vi "cont_acq_voltage_ext.vi"() -> ()   [LabVIEW 2017]
doc: "I. Description:\nThis example demonstrates how to acquire a continuous amount of data (Waveform) using an external sample clock, started by a digital edge.\n\nII. Instructions for Running:\n1. Select the physical channel to correspond to where your signal is input on the DAQ device.\n2. Enter the minimum and maximum voltage ranges.\nNote: For better accuracy try to match the Input Ranges to the expected voltage level of the measured signal.\n3. Select a source for the sample clock.\n4. Set the approximate Rate of the external clock. This allows the internal characteristics of the acquisition to be as efficient as possible. Also set the Samples to Read control. This will determine how many samples are read each time the while loop iterates. This also determines how many points are plotted on the graph each iteration.\n5. Select a source for the digital edge start trigger.\n6. Select the edge, rising or falling, on which to trigger.\n\nIII. Block Diagram Steps:\n1. Create an analog input voltage channel.\n2. Define the parameters for an External Clock Source. Additionally, define the sample mode to be continuous. The external clock rate is given to allow the internal characteristics of the acquisition to be as efficient as possible. \n3. Set the parameters for a digital edge start trigger.\n4. Call the Start VI to start the acquisition.\n5. Read the waveform data in a loop until the user hits the stop button or an error occurs.\nNote: This example reads data from one or more channels and returns an array of data. Use the Index Array function to access an individual channel of data.\n6. Call the Clear Task VI to clear the Task.\n7. Use the popup dialog box to display an error or warning if any.\n\nIV. I/O Connections Overview:\nMake sure your signal input terminal matches the Physical Channel I/O control. Also, make sure your external clock terminal matches the Clock Source Control. Finally, make sure that your digital trigger signal is connected to the terminal specified in Trigger Source. For further connection information, refer to your hardware reference manual."
uses:
  <vilib>/Utility/error.llb/DialogType.ctl
  <vilib>/DAQmx/read.llb/DAQmx Read (Analog 1D Wfm NChan NSamp).vi
  <vilib>/DAQmx/create/channels.llb/DAQmx Create Channel (AI-Voltage-Basic).vi
  <vilib>/DAQmx/configure/timing.llb/DAQmx Timing (Sample Clock).vi
  <vilib>/DAQmx/configure/trigger.llb/DAQmx Start Trigger (Digital Edge).vi
  <vilib>/DAQmx/miscellaneous.llb/DAQmx Fill In Error Info.vi
panel:
  in  "Samples to Read":i32=1000
  in  "Trigger Edge":i32(ring)=10280 items=["Rising"=10280, "Falling"=10171]
  in  "Trigger Source":tag="/Dev1/PFI0"
  in  "Maximum Value":dbl=10.0 format="%0.2f"
  in  "Minimum Value":dbl=-10.0 format="%0.2f"
  in  "Physical Channel":tag="Dev1/ai0"
  in  "Rate":dbl=10000.0 caption="Sample Rate (Hz)" format="%0.2f"
  in  "Clock Source":tag="/Dev1/PFI7"
  in  "stop":bool
  out "Measurement":waveform(dbl)[](graph)
  # "For instructions, select Help>>Show Context Help"
  # "Channel Parameters"
  # "Timing Parameters"
  # "Trigger Parameters"
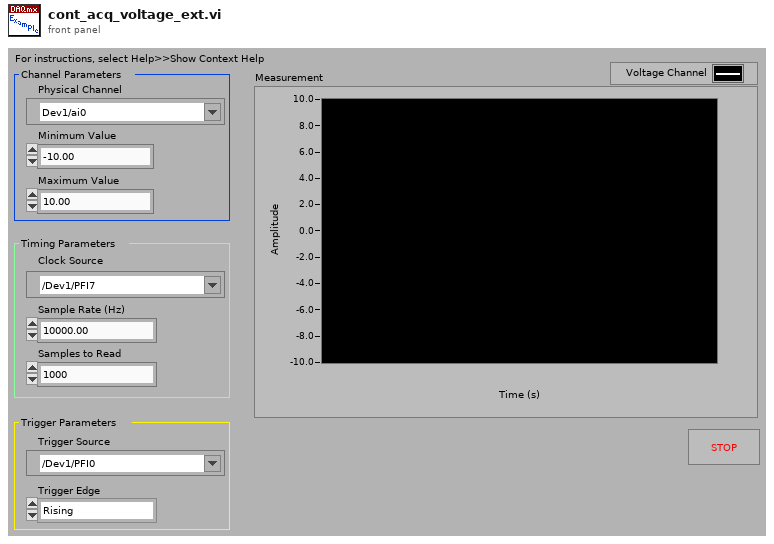
[diagram p1: front panel]
types:
  T1 = typedef "DialogType.ctl" = u16
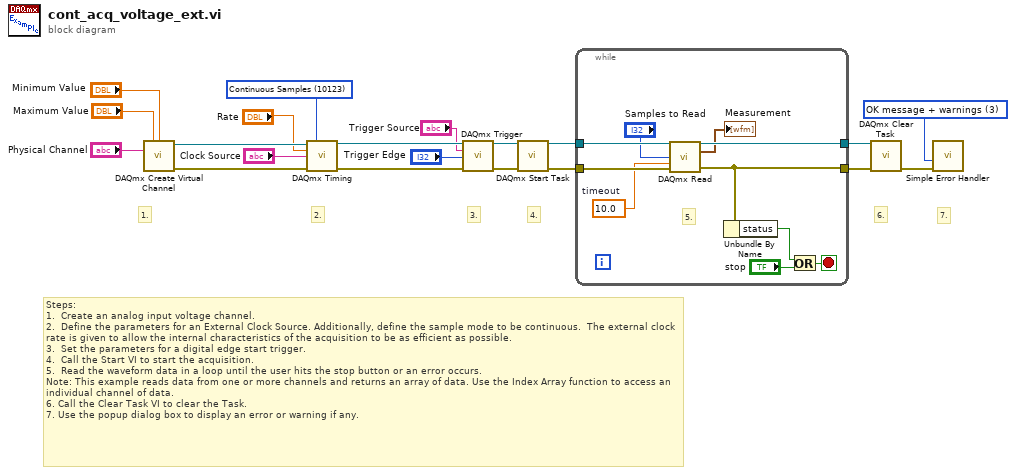
[diagram p0: block diagram]
diagram:
  w3 = T1 3 items=["no dialog", "OK message", "continue or stop message", "OK message + warnings", "continue/stop + warnings"] ("type of dialog (OK msg:1)")
  w7 = 10123 items=["Finite Samples"=10178, "Continuous Samples"=10123] ("sample mode")
  # "7."
  # "Steps: \n1.  Create an analog input voltage channel.\n2.  Define the parameters for an External Clock Source. Additionally, define the sample mode to be continuous.  The external clock rate is given to allow the internal characteristics of the acquisition to be as efficient as possible.  \n3.  Set the parameters for a digital edge start trigger.\n4.  Call the Start VI to start the acquisition.\n5.  Read the waveform data in a loop until the user hits the stop button or an error occurs.\nNote: This example reads data from one or more channels and returns an array of data. Use the Index Array function to access an individual channel of data.\n6. Call the Clear Task VI to clear the Task.\n7. Use the popup dialog box to display an error or warning if any."
  # "6."
  # "4."
  # "3."
  # "2."
  # "1."
  n1 = call-poly <vilib>:"DAQmx Create Virtual Channel.vi"("maximum value"="Maximum Value", "minimum value"="Minimum Value", "physical channels"="Physical Channel") -> ("task out"=w13:refnum<k21>, "error out"=w18:errorcluster)  [unwired: 11 in]
  n2 = call-poly <vilib>:"DAQmx Timing.vi"("task/channels in"=w13, "sample mode"=w7, "rate"="Rate", "source"="Clock Source", "error in"=w18) -> ("task out"=w12:refnum<k21>, "error out"=w17:errorcluster)  [unwired: 9 in]
  n3 = call-poly <vilib>:"DAQmx Trigger.vi"("task/channels in"=w12, "source"="Trigger Source", "edge"="Trigger Edge", "error in"=w17) -> ("task out"=w11:refnum<k21>, "error out"=w16:errorcluster)  [unwired: 10 in]
  n4 = call <vilib>:"DAQmx Start Task.vi"("task/channels in"=w11, "error in"=w16) -> ("task out"=w10:refnum<k21>, "error out"=w15:errorcluster)  [unwired: 12 in]
  n5 = while {
    tunnel: w15 -> [w30]
    tunnel: [w26] -> w1
    tunnel: w10 -> [w25]
    tunnel: [w24] -> w2
    stop <- w29 stop-if-true
    w22 = 10.0  # timeout
    # "5."
    n6 = call-poly <vilib>:"DAQmx Read.vi"("task/channels in"=w25, "number of samples per channel"="Samples to Read", "timeout"=w22, "error in"=w30) -> ("task out"=w24:refnum<k21>, "data"=→"Measurement":waveform(dbl)[], "error out"=w26:errorcluster)  [unwired: 9 in]
    n7 = Unbundle By Name(w26) -> ("status"=w27:bool)
    n8 = Or(x=w27, y="stop") -> (x .or. y?=w29:bool)
  }
  n9 = call <vilib>:"DAQmx Clear Task.vi"("task in"=w2, "error in"=w1) -> ("error out"=w14:errorcluster)  [unwired: 13 in]
  n10 = call <vilib>:"Simple Error Handler.vi"("type of dialog (OK msg:1)"=w3, "error in (no error)"=w14) -> ()  [unwired: 3 in, 5 out]
